vi "classes array.vi"() -> (0 "MBs":refnum<class "Modbus Master CR.lvclass">[](array[class]))   [LabVIEW 2021, in "Modbus Master CR.lvclass"]
uses:
  Modbus Master CR.lvclass
  ET7000/ICPCON ET-7051/ICPCON ET-7051.lvclass
  D:/my_projects/projects/Algorithms/Labview/21/Modbus_v121c/Network Protocol/MB/Modbus Master CR.lvclass
  ET7000/ICPCON ET-7042/ICPCON ET-7042.lvclass
  ET7000/ICPCON ET-7028/ICPCON ET-7028.lvclass
  ET7000/ICPCON ET-7024/ICPCON ET-7024.lvclass
  ET7000/ICPCON ET-7018i/ICPCON ET-7018i.lvclass
  ET7000/stub/stub.lvclass
  M7000/ICPCON M-7024/ICPCON M-7024.lvclass
  ET7000/TEST/TEST.lvclass
  ET7000/ICPCON ET-7017-10/ICPCON ET-7017-10.lvclass
  ET7000/ICPCON ET-7018/ICPCON ET-7018.lvclass
  Modbus Master CR.lvclass/Modbus Master CR.ctl
  ET7000/TEST1/TEST1.lvclass
  D:/my_projects/projects/Algorithms/Labview/21/Modbus_v121c/Network Protocol/ET7000/TCP/TCP.lvclass
  D:/my_projects/projects/Algorithms/Labview/21/Modbus_v121c/Network Protocol/Network Master/Network Master.lvclass
  D:/my_projects/projects/Algorithms/Labview/21/Modbus_v121c/Network Protocol/Network Protocol.lvclass
  D:/my_projects/projects/Algorithms/Labview/21/Modbus_v121c/Network Protocol/ET7000/stub/stub.lvclass
  D:/my_projects/projects/Algorithms/Labview/21/Modbus_v121c/Network Protocol/ET7000/TEST/TEST.lvclass
  D:/my_projects/projects/Algorithms/Labview/21/Modbus_v121c/Network Protocol/ET7000/TEST1/TEST1.lvclass
  D:/my_projects/projects/Algorithms/Labview/21/Modbus_v121c/Network Protocol/ET7000/ICPCON ET-7017-10/ICPCON ET-7017-10.lvclass
  D:/my_projects/projects/Algorithms/Labview/21/Modbus_v121c/Network Protocol/ET7000/ICPCON ET-7018/ICPCON ET-7018.lvclass
  D:/my_projects/projects/Algorithms/Labview/21/Modbus_v121c/Network Protocol/ET7000/ICPCON ET-7018i/ICPCON ET-7018i.lvclass
  D:/my_projects/projects/Algorithms/Labview/21/Modbus_v121c/Network Protocol/ET7000/ICPCON ET-7024/ICPCON ET-7024.lvclass
  D:/my_projects/projects/Algorithms/Labview/21/Modbus_v121c/Network Protocol/ET7000/ICPCON ET-7028/ICPCON ET-7028.lvclass
  D:/my_projects/projects/Algorithms/Labview/21/Modbus_v121c/Network Protocol/ET7000/ICPCON ET-7042/ICPCON ET-7042.lvclass
  D:/my_projects/projects/Algorithms/Labview/21/Modbus_v121c/Network Protocol/ET7000/ICPCON ET-7051/ICPCON ET-7051.lvclass
  D:/my_projects/projects/Algorithms/Labview/21/Modbus_v121c/Network Protocol/M7000/Serial/Serial.lvclass
  D:/my_projects/projects/Algorithms/Labview/21/Modbus_v121c/Network Protocol/M7000/ICPCON M-7024/ICPCON M-7024.lvclass
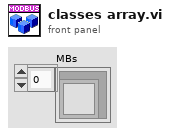
[diagram p1: front panel]
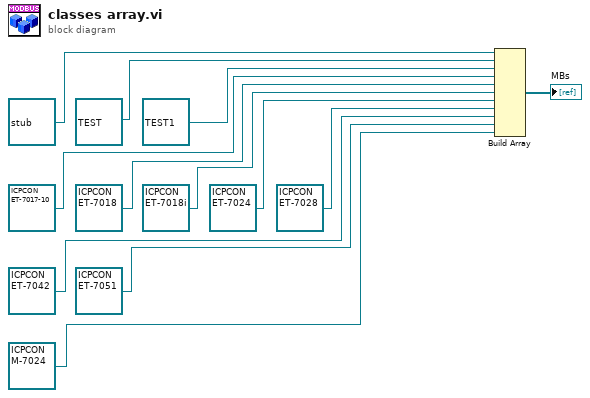
[diagram p0: block diagram]
diagram:
  n1 = Build Array(refnum<class "stub.lvclass"> refnum ("stub.lvclass"), refnum<class "TEST.lvclass"> refnum ("TEST.lvclass"), refnum<class "TEST1.lvclass"> refnum ("TEST1.lvclass"), refnum<class "ICPCON ET-7017-10.lvclass"> refnum ("ICPCON ET-7017-10.lvclass"), refnum<class "ICPCON ET-7018.lvclass"> refnum ("ICPCON ET-7018.lvclass"), refnum<class "ICPCON ET-7018i.lvclass"> refnum ("MB_v2.lvlib:ICPCON ET-7018i.lvclass"), refnum<class "ICPCON ET-7024.lvclass"> refnum ("MB_v2.lvlib:ICPCON ET-7024.lvclass"), refnum<class "ICPCON ET-7028.lvclass"> refnum ("MB_v2.lvlib:ICPCON ET-7028.lvclass"), refnum<class "ICPCON ET-7042.lvclass"> refnum ("MB_v2.lvlib:ICPCON ET-7042.lvclass"), refnum<class "ICPCON ET-7051.lvclass"> refnum ("MB_v2.lvlib:ICPCON ET-7051.lvclass"), refnum<class "ICPCON M-7024.lvclass"> refnum ("ICPCON M-7024.lvclass")) -> (→"MBs":refnum<class "Modbus Master CR.lvclass">[])
